vi "Read TDMS Wavenames into Ring.vi"(8 "error in (no error)":errorcluster, 9 "Ring Refs []":refnum<vi>[](array[refnum]), 10 "File or Folder Path":path=path "C:/", 11 "LVtoITX.lvclass":refnum<class "LV to ITX.lvclass">) -> (0 "error out":errorcluster, 3 "LVtoITX.lvclass out":refnum<class "LV to ITX.lvclass">)   [LabVIEW 2016, in "LV to ITX.lvclass"]
uses:
  LV to ITX.lvclass
panel:
  out "Names []":string[](array[string])
  out "Channels":cluster{"X":u16, "Y":u16, "N":u16} {"N" items=["time", "temp", "B", "AI1", "AI2", "AI3", "AI4", "AI5", "AI6", "AO1", "AO2", "AO3", "AO4"]; "Y" items=["time", "temp", "B", "AI1", "AI2", "AI3", "AI4", "AI5", "AI6", "AO1", "AO2", "AO3", "AO4"]; "X" items=["time", "temp", "B", "AI1", "AI2", "AI3", "AI4", "AI5", "AI6", "AO1", "AO2", "AO3", "AO4"]}
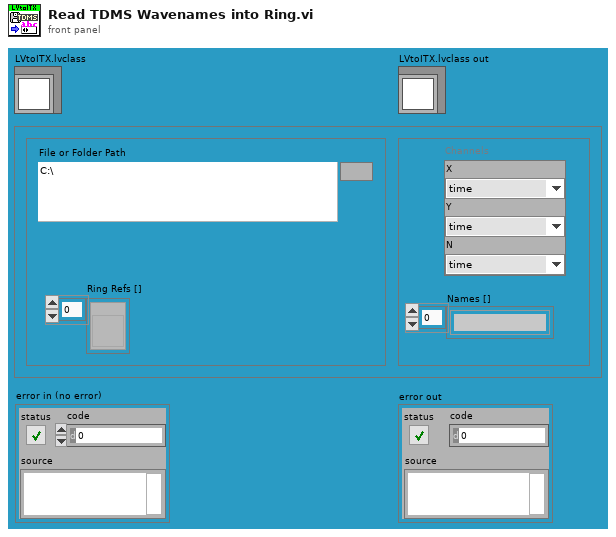
[diagram p1: front panel]
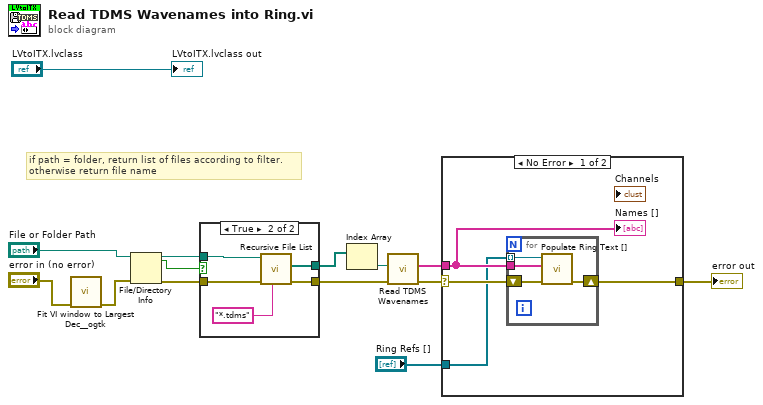
[diagram p0: block diagram]
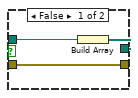
[diagram p3: hidden frame]
diagram:
  # "if path = folder, return list of files according to filter.\notherwise return file name"
  n1 = call <userlib>:"Fit VI window to Largest Dec__ogtk.vi"("error in (no error)"="error in (no error)") -> ("error out"=w7:errorcluster)  [unwired: 5 in, 1 out]
  n2 = File/Directory Info(path="File or Folder Path", error in=w7) -> (path out=w10:path, directory=w12:bool, error out=w11:errorcluster)  [unwired: 4 out]
  n3 = case shown="True" w12 {
    tunnel: [w17 w21] -> w2
    tunnel: w10 -> [w16 w22]
    tunnel: w11 -> [w15 w20]
    tunnel: [w15 w19] -> w13
    frame False {
      n4 = Build Array(w16) -> (w17:path[])
    }
    frame True {
      n5 = call <vilib>:"Recursive File List.vi"("pattern"="*.tdms", "error in (no error)"=w20, "Folder Path"=w22) -> ("error out"=w19:errorcluster, "All Files in Dir"=w21:path[])  [unwired: 4 in, 3 out]
    }
  }
  n6 = Index Array(array=w2) -> (element=w6:path)  [unwired: 1 in]
  n7 = call "Read TDMS Wavenames.vi"("error in (no error)"=w13, "path"=w6) -> ("error out"=w4:errorcluster, "Wavenames"=w5:string[])  [unwired: 7 in, 1 out]
  n8 = case shown="No Error" w4 {
    selector: w4 -> [w26 w31]
    tunnel: w5 -> [w25 _]
    tunnel: [w24 w31] -> w3
    tunnel: "Ring Refs []" -> [w23 _]
    frame No Error {
      n9 = for {
        tunnel: w25 -> [w29]
        shift-right: [w28] -> w24
        shift-left: w26 -> [w30]
        tunnel: w23 -> [w27] mode=indexing
        n10 = call "Populate Ring Text [].vi"("error in (no error)"=w30, "Strings []"=w29, "Ring in"=w27) -> ("error out"=w28:errorcluster)  [unwired: 8 in]
      }
      "Names []" <- w25
    }
    frame Error {
    }
  }
  "error out" <- w3
  "LVtoITX.lvclass out" <- "LVtoITX.lvclass"
